vi "Actor.vi"(8 "error in (no error)":errorcluster, 9 "queue out":refnum<queue>, 10 "Caller_Queue":refnum<queue>, 11 "Actor Input":refnum<class "Counter.lvclass">) -> (0 "error out":errorcluster)   [LabVIEW 2018, in "Counter.lvclass"]
uses:
  Counter Class/Counter.lvclass
  Message Class/Message.lvclass
  Counter Class/Counter.lvclass/Counter.ctl
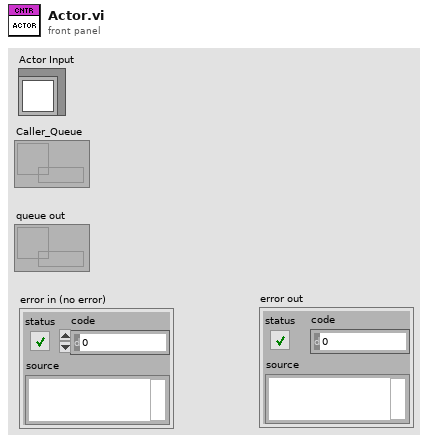
[diagram p1: front panel]
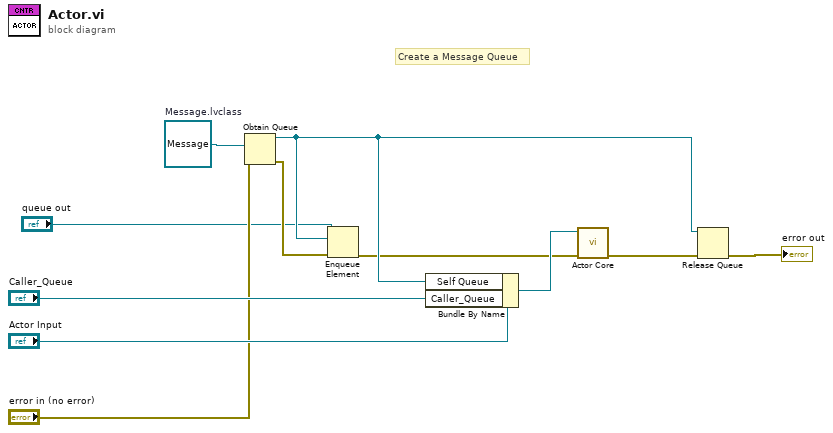
[diagram p0: block diagram]
diagram:
  w11 = refnum<class "Message.lvclass"> refnum  # Message.lvclass
  # "Create a Message Queue"
  n1 = Obtain Queue(element data type=w11, error in (no error)="error in (no error)") -> (queue out=w5:refnum<queue>, error out=w4:errorcluster)  [unwired: 3 in, 1 out]
  n2 = Enqueue Element(queue="queue out", element=w5, error in (no error)=w4) -> (error out=w3:errorcluster)  [unwired: 1 in, 2 out]
  n3 = Bundle By Name(cluster="Actor Input", "Self Queue"=w5, "Caller_Queue"="Caller_Queue") -> (w6:refnum<class "Counter.lvclass">)
  n4 = call "Actor Core.vi"("error In"=w3, "Counter.lvclass"=w6) -> ("error out"=w10:errorcluster)  [unwired: 8 in, 1 out]
  n5 = Release Queue(queue=w5, error in (no error)=w10) -> (error out=→"error out":errorcluster)  [unwired: 1 in, 2 out]
